vi "_openVIOnTarget.vi"(8 "error in (no error)":errorcluster, 9 "VI Path":string, 10 "Target Name":string, 11 "Project Path":string) -> (0 "error out":errorcluster, 3 "VI Reference":refnum<vi>)   [LabVIEW 2014, in "tWorkerCommandRunner.lvlib" / "tWorkerCommandRunner.lvclass"]
doc: "Returns a reference to a specified VI located under a specified target in a specified project."
uses:
  tWorkerCommandRunner.lvclass
  <vilib>/ErrorRing/Error Ring.xnode
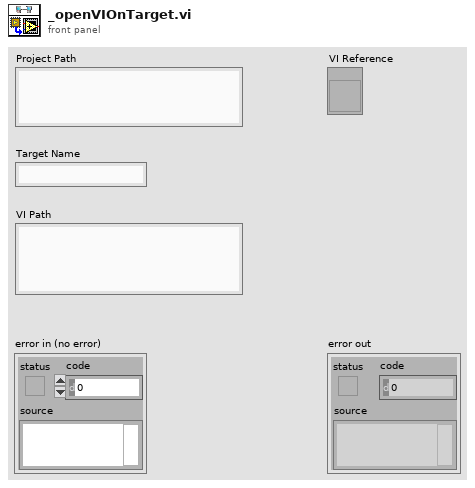
[diagram p1: front panel]
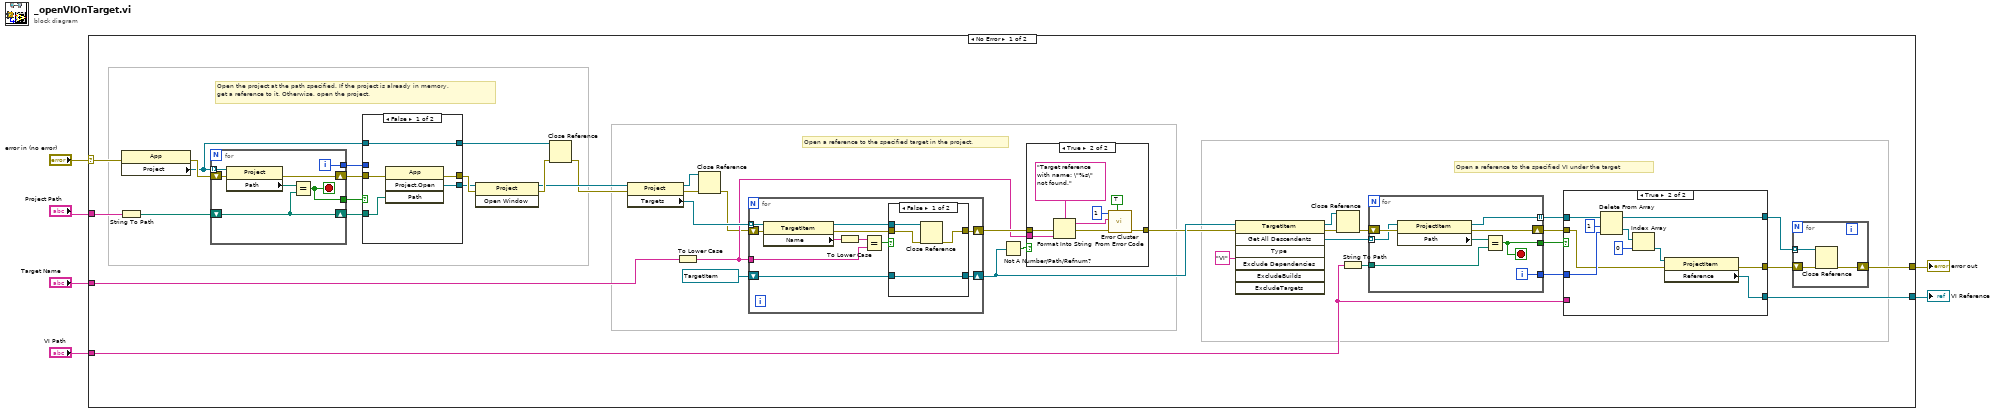
[diagram p0: block diagram]
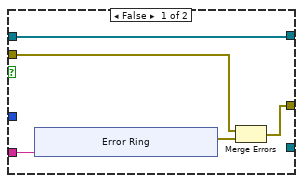
[diagram p2: hidden frame]
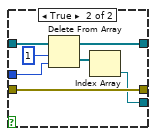
[diagram p5: hidden frame]
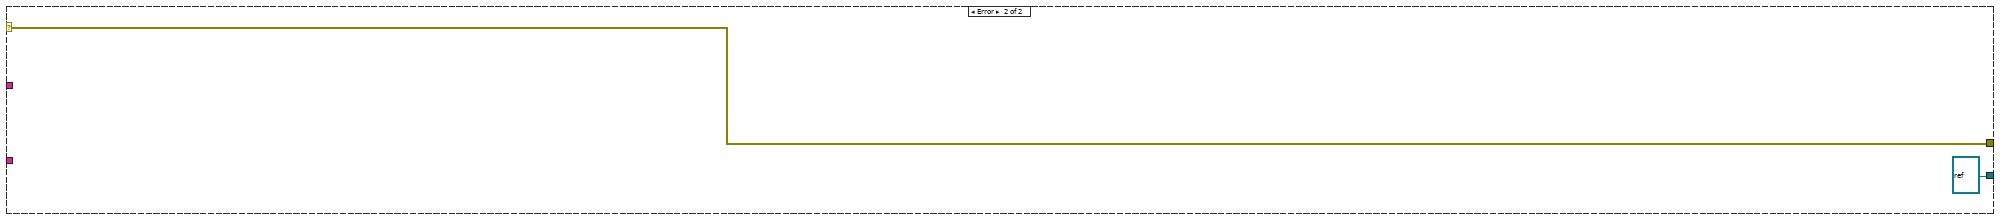
[diagram p6: hidden frame]
diagram:
  n1 = case shown="No Error" "error in (no error)" {
    selector: "error in (no error)" -> [w35 w127]
    tunnel: [w16 w127] -> w5
    tunnel: "Project Path" -> [w37 _]
    tunnel: "Target Name" -> [w27 _]
    tunnel: "VI Path" -> [w14 _]
    tunnel: [w10 refnum<vi> refnum ("Reference")] -> w1
    frame No Error {
      # "Open a reference to the specified VI under the target"
      # "Open a reference to the specified target in the project."
      # "Open the project at the path specified. If the project is already in memory,\nget a reference to it. Otherwise, open the project."
      n2 = String To Path(string=w37) -> (path=w36:path)
      n3 = property class="App"(error in=w35) -> (error out=w47:errorcluster, "Project"=w43:refnum<vi>[])  [unwired: 1 in, 1 out]
      n4 = for {
        tunnel: w43 -> [w125] mode=indexing
        tunnel: [w122] -> w45
        tunnel: [w121] -> w46
        shift-right: [w120] -> w44
        shift-left: w47 -> [w124]
        shift-right: [w119] -> w41
        shift-left: w36 -> [w119]
        i -> [w122]
        stop <- w121 stop-if-true
        n5 = property class="Project"(reference=w125, error in=w124) -> (error out=w120:errorcluster, "Path"=w123:path)  [unwired: 1 out]
        n6 = Equal?(x=w123, y=w119) -> (x = y?=w121:bool)
      }
      n7 = case shown="False" w46 {
        tunnel: w45 -> [_ w116]
        tunnel: w44 -> [w110 w113]
        tunnel: w43 -> [w111 w118]
        tunnel: [w107 w113] -> w40
        tunnel: [w108 w112] -> w39
        tunnel: [w111 w114] -> w42
        tunnel: w41 -> [w109 _]
        frame False {
          n8 = invoke class="App" method="Project.Open"(error in=w110, "Path"=w109) -> (error out=w107:errorcluster, "Project:Open"=w108:refnum<vi>)  [unwired: 2 in, 2 out]
        }
        frame True {
          n9 = Delete From Array(array=w118, length=1, index=w116) -> (deleted portion=w115:refnum<vi>[], array with subset deleted=w114:refnum<vi>[])
          n10 = Index Array(array=w115) -> (element=w112:refnum<vi>)  [unwired: 1 in]
        }
      }
      n11 = invoke class="Project" method="Open Window"(reference=w39, error in=w40) -> (reference out=w29:refnum<vi>, error out=w38:errorcluster)  [unwired: 1 in, 1 out]
      n12 = Close Reference(reference=w42, error in (no error)=w38) -> (error out=w28:errorcluster)
      n13 = property class="Project"(reference=w29, error in=w28) -> (reference out=w8:refnum<vi>, error out=w9:errorcluster, "Targets"=w34:refnum<vi>[])
      n14 = To Lower Case(string=w27) -> (all lower case string=w30:string)
      n15 = Close Reference(reference=w8, error in (no error)=w9) -> (error out=w7:errorcluster)
      n16 = for {
        tunnel: w34 -> [w100] mode=indexing
        tunnel: w30 -> [w99]
        shift-right: [w96] -> w18
        shift-left: refnum<vi> refnum ("Project Reference") -> [w95]
        shift-right: [w92] -> w31
        shift-left: w7 -> [w94]
        n17 = property class="TargetItem"(reference=w100, error in=w94) -> (reference out=w97:refnum<vi>, error out=w93:errorcluster, "Name"=w91:string)
        n18 = To Lower Case(string=w91) -> (all lower case string=w90:string)
        n19 = Equal?(x=w90, y=w99) -> (x = y?=w98:bool)
        n20 = case shown="False" w98 {
          tunnel: w97 -> [w103 w106]
          tunnel: [w104 w106] -> w96
          tunnel: w95 -> [w104 _]
          tunnel: w93 -> [w102 w105]
          tunnel: [w101 w105] -> w92
          frame False {
            n21 = Close Reference(reference=w103, error in (no error)=w102) -> (error out=w101:errorcluster)
          }
          frame True {
          }
        }
      }
      n22 = Not A Number/Path/Refnum?(number/path/refnum=w18) -> (NaN/Path/Refnum?=w32:bool)
      n23 = case shown="True" w32 {
        tunnel: w31 -> [w81 w86]
        tunnel: w30 -> [_ w88]
        tunnel: [w81 w82] -> w17
        frame False {
        }
        frame True {
          n24 = Format Into String(format string="Target reference with name: \"%s\" not found.", error in=w86, w88) -> (resulting string=w87:string, error out=w85:errorcluster)  [unwired: 1 in]
          n25 = call <vilib>:"Error Cluster From Error Code.vi"("show call chain? (False)"=TRUE, "error in (no error)"=w85, "error message (\"\")"=w87, "error code (0)"=1) -> ("error out"=w82:errorcluster)  [unwired: 5 in]
        }
      }
      n26 = invoke class="TargetItem" method="Get All Descendents"(reference=w18, error in=w17, "Type"="VI") -> (reference out=w12:refnum<vi>, error out=w13:errorcluster, "All Descendents"=w25:refnum<vi>[])  [unwired: 4 in, 4 out]
      n27 = Close Reference(reference=w12, error in (no error)=w13) -> (error out=w11:errorcluster)
      n28 = String To Path(string=w14) -> (path=w15:path)
      n29 = for {
        tunnel: w15 -> [w80]
        tunnel: w25 -> [w78] mode=indexing
        shift-right: [w74] -> w23
        shift-left: w11 -> [w79]
        tunnel: [w76] -> w21
        tunnel: [w75] -> w24
        tunnel: [w73] -> w22 mode=indexing
        i -> [w76]
        stop <- w75 stop-if-true
        n30 = property class="ProjectItem"(reference=w78, error in=w79) -> (reference out=w73:refnum<vi>, error out=w74:errorcluster, "Path"=w77:path)
        n31 = Equal?(x=w77, y=w80) -> (x = y?=w75:bool)
      }
      n32 = case shown="True" w24 {
        tunnel: w23 -> [w54 w63]
        tunnel: w22 -> [w52 w72]
        tunnel: [w53 w66] -> w19
        tunnel: w21 -> [_ w70]
        tunnel: [_ w65] -> w10
        tunnel: [w52 w64] -> w20
        tunnel: w14 -> [w51 _]
        frame False {
          n33 = xnode "Error Ring"("parameter 0"=w51) -> ("error out"=w55:errorcluster)
          n34 = Merge Errors(w54, w55) -> (w53:errorcluster)
        }
        frame True {
          n35 = Delete From Array(array=w72, length=1, index=w70) -> (deleted portion=w69:refnum<vi>[], array with subset deleted=w64:refnum<vi>[])
          n36 = Index Array(array=w69, index=0) -> (element=w67:refnum<vi>)
          n37 = property class="ProjectItem"(reference=w67, error in=w63) -> (error out=w66:errorcluster, "Reference"=w65:refnum<vi>)  [unwired: 1 out]
        }
      }
      n38 = for {
        tunnel: w20 -> [w49] mode=indexing
        shift-right: [w48] -> w16
        shift-left: w19 -> [w50]
        n39 = Close Reference(reference=w49, error in (no error)=w50) -> (error out=w48:errorcluster)
      }
    }
    frame Error {
    }
  }
  "error out" <- w5
  "VI Reference" <- w1
